vi "SCLN_ClientConnected.vi"(1 "Server Name":string) -> (0 "Connected":bool)   [LabVIEW 2015]
uses:
  SCLN_RW_Select.ctl
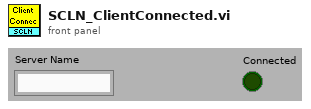
[diagram p1: front panel]
types:
  T1 = typedef "SCLN_RW_Select.ctl" = enum16{"Read", "Write"}
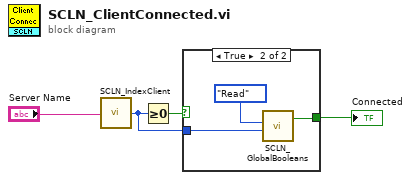
[diagram p0: block diagram]
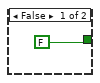
[diagram p2: hidden frame]
diagram:
  n1 = call "SCLN_IndexClient.vi"("Server Name"="Server Name") -> ("Index"=w2:i32)
  n2 = Greater Or Equal To 0?(x=w2) -> (x >= 0?=w1:bool)
  n3 = case shown="True" w1 {
    tunnel: [FALSE w7] -> w3
    tunnel: w2 -> [_ w6]
    frame False {
    }
    frame True {
      n4 = call "SCLN_GlobalBooleans.vi"("Element"=w6, "Operation"=SCLN_RW_Select."Read" ("GBL_RW")) -> ("Read Value"=w7:bool)  [unwired: 2 in, 1 out]
    }
  }
  "Connected" <- w3
